vi "HDF5 Read and Write.vi"() -> ()   [LabVIEW 2016]
doc: "This example demonstrates how to write and read a simple dataset. Experiment by changing \"Data to write\" and \"Data read\" to any datatype or array of datatype supported by the library. Make sure that both the control and the indicator have matching datatypes!"
uses:
  <vilib>/UPVI/lvhdf5/dataset.llb/LVH5D Operation.ctl
  <vilib>/UPVI/lvhdf5/file.llb/LVH5F Operation.ctl
  <vilib>/Utility/miscctls.llb/LVRectTypeDef.ctl
  <vilib>/UPVI/lvhdf5/group.llb/H5G_obj_t.ctl
  <vilib>/UPVI/lvhdf5/utility.llb/Select HDF5 Dialog.vi
  <vilib>/UPVI/lvhdf5/utility.llb/Select HDF5 Dialog (Object Only).vi
  <vilib>/UPVI/lvhdf5/dataset.llb/Simple H5Dwrite (Variant).vi
  <vilib>/UPVI/lvhdf5/dataset.llb/Simple H5Dread (Variant).vi
  <vilib>/UPVI/lvhdf5/dataset.llb/Simple H5Dwrite.xnode
  <vilib>/UPVI/lvhdf5/library.llb/HDF5 Ref.ctl
  <vilib>/UPVI/lvhdf5/dataset.llb/Simple H5Dread.xnode
  <vilib>/UPVI/lvhdf5/identifier.llb/Not an HDF5 Refnum Constant.vi
  <vilib>/Utility/error.llb/Error Cluster From Error Code.vi
  <vilib>/UPVI/lvhdf5/dataspace.llb/H5Sselect_hyperslab.vi
  <vilib>/UPVI/lvhdf5/dataset.llb/H5Dget_space.vi
  <vilib>/UPVI/lvhdf5/dataspace.llb/H5Sclose.vi
  <vilib>/UPVI/lvhdf5/dataset.llb/H5Dclose.vi
  <vilib>/UPVI/lvhdf5/utility.llb/Select HDF5 Dialog (File and Object).vi
  <vilib>/UPVI/lvhdf5/dataset.llb/OpenCreateReplace Dataset by Element Type.vi
  <vilib>/UPVI/lvhdf5/dataset.llb/H5Dwrite (Variant).vi
  <vilib>/UPVI/lvhdf5/attribute.llb/private/LVH5AwriteWDTAttrs.vi
  <vilib>/UPVI/lvhdf5/dataset.llb/OpenCreateReplace Dataset.vi
  <vilib>/UPVI/lvhdf5/dataspace.llb/H5Sget_simple_extent_dims.vi
  <vilib>/UPVI/lvhdf5/dataset.llb/H5Dread (Variant).vi
  <vilib>/UPVI/lvhdf5/attribute.llb/private/LVH5AreadWDTAttrs.vi
panel:
  in  "Operation":enum32{"Write", "Read"}(tab)
  in  "Data to write":dbl[](array[numeric])=[2.2, 4.4, 3.3, 5.5, 6.6]
  out "Data read":dbl[](array[numeric])
  in  "Dataset name":string="test"
  in  "File path":path=path "Test.hdf5"
  # "See VI and block diagram documentation"
  # "LVHDF5 Example VI\nCopyright (c) 2014 UPVI, LLC\nwww.upvi.net\n\nThis VI is exempt from the LVHDF5 license and may be freely copied, modified, distributed or incorporated into other applications."
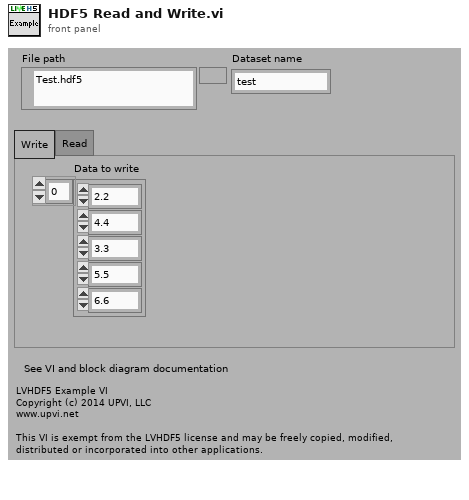
[diagram p1: front panel]
types:
  T1 = typedef "LVH5F Operation.ctl" = enum16{"open", "open or create", "create or replace", "create or replace (with confirmation)", "create", "open (read only)"}
  T2 = typedef "LVH5D Operation.ctl" = enum16{"open", "replace", "create", "open or create", "create or replace", "create or replace with confirmation"}
  T3 = typedef "LVRectTypeDef.ctl" = cluster{"Left":i16, "Top":i16, "Right":i16, "Bottom":i16}
  T4 = cluster{"Behavior":enum32{"Invalid", "Default", "Floating", "Floating/Auto-Hide", "Modal"}, "Position":T3, "Center":bool, "Title":string}
  T5 = typedef "H5G_obj_t.ctl" = i32
  T6 = cluster{"Object Types (any)":T5[], "Object Pattern":string}
  T7 = typedef "HDF5 Ref.ctl" = refnum<k1>
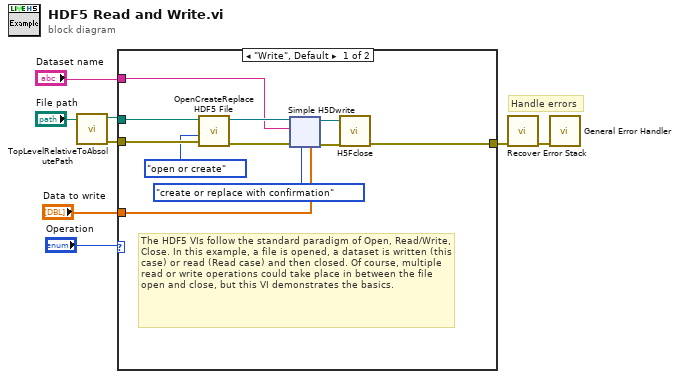
[diagram p0: block diagram]
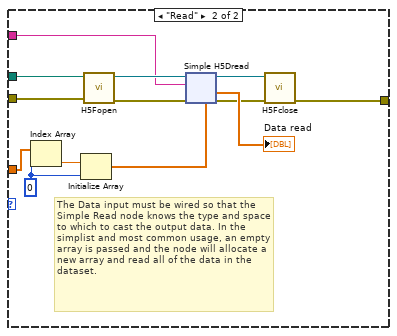
[diagram p2: hidden frame]
diagram:
  # "Handle errors"
  n1 = call "TopLevelRelativeToAbsolutePath.vi"("Path Relative to Top Level VI"="File path") -> ("error out"=w3:errorcluster, "Absolute path"=w4:path)  [unwired: 9 in]
  n2 = case shown="\"Write\", Default" "Operation" {
    tunnel: w4 -> [w19 w234]
    tunnel: "Data to write" -> [w16 w230]
    tunnel: "Dataset name" -> [w9 w223]
    tunnel: w3 -> [w15 w226]
    tunnel: [w10 w224] -> w2
    frame "Write", Default {
      # "The HDF5 VIs follow the standard paradigm of Open, Read/Write, Close. In this example, a file is opened, a dataset is written (this case) or read (Read case) and then closed. Of course, multiple read or write operations could take place in between the file open and close, but this VI demonstrates the basics."
      n3 = call <vilib>:"OpenCreateReplace HDF5 File.vi"("error in (no error)"=w15, "function (open or create)"=LVH5F_Operation."open or create", "path"=w19) -> ("error out"=w18:errorcluster, "HDF5 Ref out"=w14:T7)  [unwired: 5 in]
      n4 = xnode "Simple H5Dwrite"("Dataset Path"=w9, "error in (no error)"=w18, "operation (open or create)"=LVH5D_Operation."create or replace with confirmation", "HDF5 Path or Ref"=w14, "Data"=w16) -> ("HDF5 Ref out"=w11:T7, "error out"=w17:errorcluster)  [unwired: 3 in, 1 out]
      n5 = call <vilib>:"H5Fclose.vi"("error in (no error)"=w17, "HDF5 Ref"=w11) -> ("error out"=w10:errorcluster)  [unwired: 7 in]
    }
    frame "Read" {
      w228 = 0 ("index")
      # "The Data input must be wired so that the Simple Read node knows the type and space to which to cast the output data. In the simplist and most common usage, an empty array is passed and the node will allocate a new array and read all of the data in the dataset."
      n6 = Index Array(array=w230, index=w228) -> (element=w229:dbl)
      n7 = Initialize Array(w229, w228) -> (w227:dbl[])
      n8 = call <vilib>:"H5Fopen.vi"("error in (no error)"=w226, "path"=w234) -> ("error out"=w233:errorcluster, "HDF5 Ref out"=w225:T7)  [unwired: 6 in]
      n9 = xnode "Simple H5Dread"("Dataset Path"=w223, "error in (no error)"=w233, "HDF5 Path or Ref"=w225, "Data"=w227) -> ("HDF5 Ref out"=w222:T7, "error out"=w231:errorcluster, "Data out"=→"Data read":dbl[])  [unwired: 1 out]
      n10 = call <vilib>:"H5Fclose.vi"("error in (no error)"=w231, "HDF5 Ref"=w222) -> ("error out"=w224:errorcluster)  [unwired: 7 in]
    }
  }
  n11 = call <vilib>:"Recover Error Stack.vi"("error in (no error)"=w2) -> ("error out"=w1:errorcluster)  [unwired: 5 in, 3 out]
  n12 = call <vilib>:"General Error Handler.vi"("error in (no error)"=w1) -> ()  [unwired: 10 in, 5 out]
